vi "reporte 8 B.vi"() -> ()   [LabVIEW 2015]
panel:
  out "Discriminante < 0":bool
  out "Discriminante = 0":bool
  out "Discriminante > 0":bool
  out "Discriminante":dbl
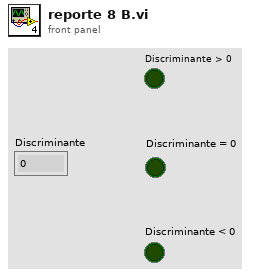
[diagram p1: front panel]
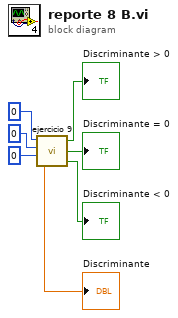
[diagram p0: block diagram]
diagram:
  n1 = call "ejercicio 9.vi"("Número C"=0, "Número A"=0, "Número B"=0) -> ("Discriminante < 0"=→"Discriminante < 0":bool, "Discriminante = 0"=→"Discriminante = 0":bool, "Discriminante > 0"=→"Discriminante > 0":bool, "Discriminante"=→"Discriminante":dbl)
